vi "Example-超声波测距-uart.vi"() -> ()   [LabVIEW 2018]
uses:
  c8864175-e948-409a-9e2f-56297bfabe3e.vi
panel:
  in  "Voltage(V)":dbl=5.0 format="%#_13g"
  out "ret":i32[](array[numeric])
  in  "停止":bool
  in  "Write":bool
  in  "loop":i32=100
  out "数值":i32
  out "历史数据":dbl(graph)
  out "SerialNumber":string
  out "rxcount out":i32
  out "rgRX":u8[](array[numeric])
  in  "Tx data":u8[](array[numeric])=[253, 0, 204, 223] format="%.0x"
  in  "RX IO(0~15)":i32=1
  in  "TX IO(0~15)":i32
  in  "Frequency(Hz)":i32(ring)=9600 items=["110"=110, "150"=150, "300"=300, "600"=600, "1200"=1200, "2400"=2400, "4800"=4800, "9600"=9600, "14400"=14400, "19200"=19200, "28800"=28800, "38400"=38400, "56000"=56000, "57600"=57600, "115200"=115200, "128000"=128000, "153600"=153600, "230400"=230400, "256000"=256000, "406800"=406800, "921600"=921600]
  out "returns":i32[](array[numeric])
  out "error out":errorcluster caption="错误输出"
  in  "error in (no error)":errorcluster caption="错误输入（无错误）"
  out "ftHandle out":u64=363562184
  in  "设备索引":i32
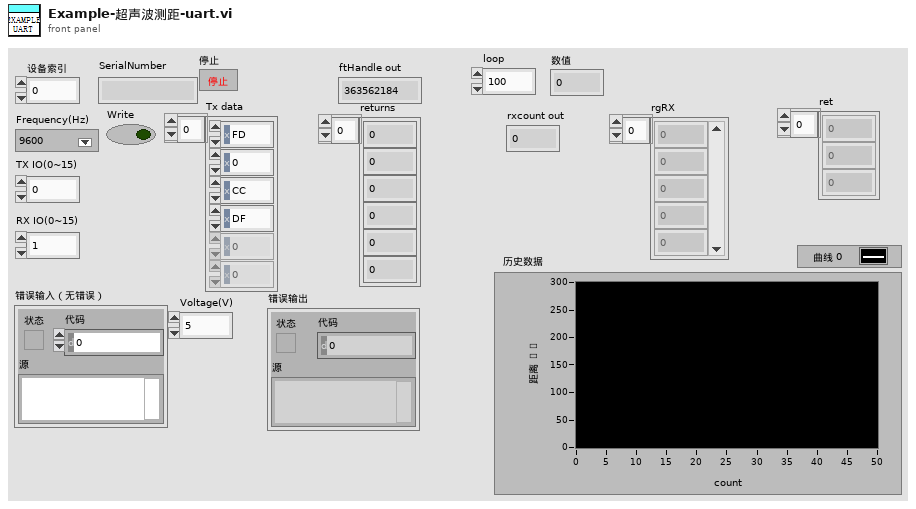
[diagram p1: front panel]
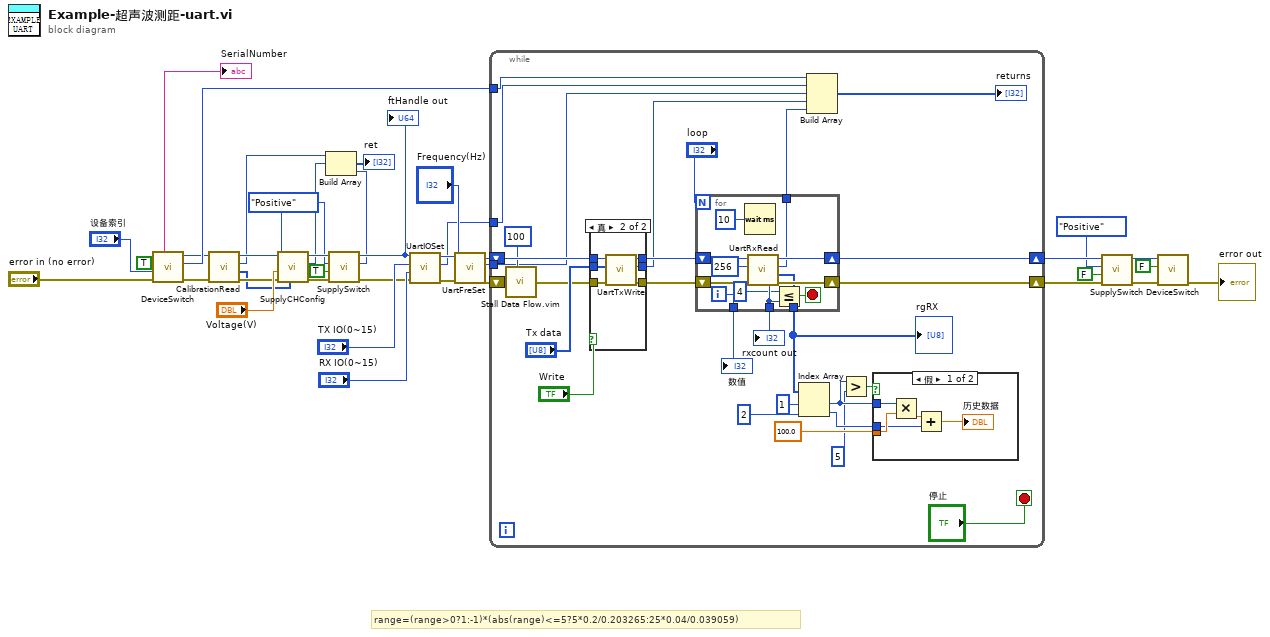
[diagram p0: block diagram]
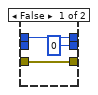
[diagram p3: hidden frame]
diagram:
  w18 = enum16{"Positive", "Negative"}."Positive" ("CH")
  # "range=(range>0?1:-1)*(abs(range)<=5?5*0.2/0.203265:25*0.04/0.039059)"
  n1 = call "DeviceSwitch.vi"("error in (no error)"="error in (no error)", "Device Index"="设备索引", "Open"=TRUE) -> ("error out"=w9:errorcluster, "function return"=w25:i32, "handle out"=w6:u64, "SerialNumber"=→"SerialNumber":string)  [unwired: 4 in, 1 out]
  n2 = call "CalibrationRead.vi"("handle"=w6, "error in (no error)"=w9) -> ("handle out"=w7:u64, "function return"=w4:i32, "CalArray"=w5:u8[], "error out"=w8:errorcluster)  [unwired: 5 in]
  n3 = call "SupplyCHConfig.vi"("CalArray"=w5, "error in (no error)"=w8, "Voltage(V)"="Voltage(V)", "CH"=w18, "handle"=w7) -> ("error out"=w19:errorcluster, "function return"=w3:i32, "handle out"=w21:u64)  [unwired: 3 in, 1 out]
  n4 = call "SupplySwitch.vi"("error in (no error)"=w19, "Output"=TRUE, "CH"=w18, "handle"=w21) -> ("error out"=w17:errorcluster, "function return"=w2:i32, "handle out"=w20:u64)  [unwired: 5 in]
  "ftHandle out" <- w20
  n5 = Build Array(w4, w3, w2) -> (→"ret":i32[])
  n6 = call "UartIOSet.vi"("error in (no error)"=w17, "RX IO(0~15)"="RX IO(0~15)", "TX IO(0~15)"="TX IO(0~15)", "handle"=w20) -> ("error out"=w35:errorcluster, "function return"=w24:i32, "handle out"=w31:u64)  [unwired: 5 in]
  n7 = call "UartFreSet.vi"("error in (no error)"=w35, "Frequency(Hz)"="Frequency(Hz)", "handle"=w31) -> ("error out"=w29:errorcluster, "function return"=w23:i32, "handle out"=w30:u64)  [unwired: 6 in]
  n8 = while {
    shift-right: [w62] -> w13
    shift-left: w30 -> [w66]
    shift-right: [w63] -> w15
    shift-left: w29 -> [w64]
    tunnel: w25 -> [w54]
    tunnel: w24 -> [w53]
    tunnel: w23 -> [w52]
    stop <- "停止" stop-if-true
    n9 = call "Stall Data Flow.vim"("value in"=w64, "milliseconds to wait"=u32 100) -> ("value out"=w58:errorcluster)  [unwired: 1 out]
    n10 = case shown="真" "Write" {
      tunnel: w66 -> [w86 w92]
      tunnel: "Tx data" -> [_ w91]
      tunnel: w58 -> [w84 w90]
      tunnel: [0 ("function return") w89] -> w51
      tunnel: [w84 w88] -> w61
      tunnel: [w86 w87] -> w60
      frame False {
      }
      frame True {
        n11 = call "UartTxWrite.vi"("error in (no error)"=w90, "data"=w91, "handle"=w92) -> ("error out"=w88:errorcluster, "function return"=w89:i32, "handle out"=w87:u64)  [unwired: 6 in]
      }
    }
    n12 = for {
      N: "loop" -> [_]
      tunnel: [w79] -> w50
      tunnel: [w78] -> w45
      tunnel: [w77] -> w49
      shift-right: [w82] -> w63
      shift-left: w61 -> [w83]
      shift-right: [w81] -> w62
      shift-left: w60 -> [w80]
      tunnel: [w74] -> w47
      i -> [w74]
      stop <- w76 stop-if-true
      n13 = Wait (ms)(milliseconds to wait=u32 10 ("等待时间（毫秒）")) -> ()  [unwired: 1 out]
      n14 = call "UartRxRead.vi"("error in (no error)"=w83, "length"=256, "handle"=w80) -> ("error out"=w82:errorcluster, "rgRX"=w78:u8[], "function return"=w79:i32, "handle out"=w81:u64, "rxcount out"=w77:i32)  [unwired: 4 in]
      n15 = Less Or Equal?(x=4, y=w77) -> (x <= y?=w76:bool)
    }
    "rgRX" <- w45
    "rxcount out" <- w49
    "数值" <- w47
    n16 = Index Array(array=w45, index #1=1 ("索引"), index #2=2 ("索引")) -> (element #1=w41:u8, element #2=w42:u8)
    n17 = Build Array(w54, w53, w52, w51, w50) -> (→"returns":i32[])
    n18 = Greater?(x=w41, y=u8 5) -> (0:w39:bool)
    n19 = case shown="假" w39 {
      tunnel: 100.0 ("y") -> [w69 _]
      tunnel: w42 -> [w68 _]
      tunnel: w41 -> [w67 _]
      frame False {
        n20 = Multiply(x=w67, y=w69) -> (x*y=w70:dbl)
        n21 = Add(x=w70, y=w68) -> (x+y=→"历史数据":dbl)
      }
      frame True {
      }
    }
  }
  n22 = call "SupplySwitch.vi"("error in (no error)"=w15, "Output"=FALSE, "CH"=enum16{"Positive", "Negative"}."Positive", "handle"=w13) -> ("error out"=w14:errorcluster, "handle out"=w12:u64)  [unwired: 5 in, 1 out]
  n23 = call "DeviceSwitch.vi"("error in (no error)"=w14, "Open"=FALSE, "handle"=w12) -> ("error out"=→"error out":errorcluster)  [unwired: 4 in, 4 out]
